vi "Load FIR coeff from CSV.vi"(8 "error in (no error)":T1, 11 "Path":path) -> (0 "error out":T1, 2 "valid":bool, 3 "1D Array":cdb[](array[numeric]))   [LabVIEW 2019]
uses:
  <vilib>/Utility/file.llb/Read Delimited Spreadsheet (string).vi
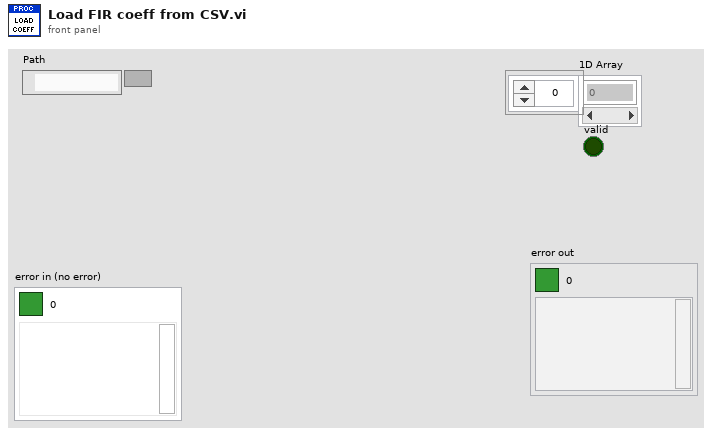
[diagram p1: front panel]
types:
  T1 = cluster{"Boolean Round":bool, "code":i32, "source":string}
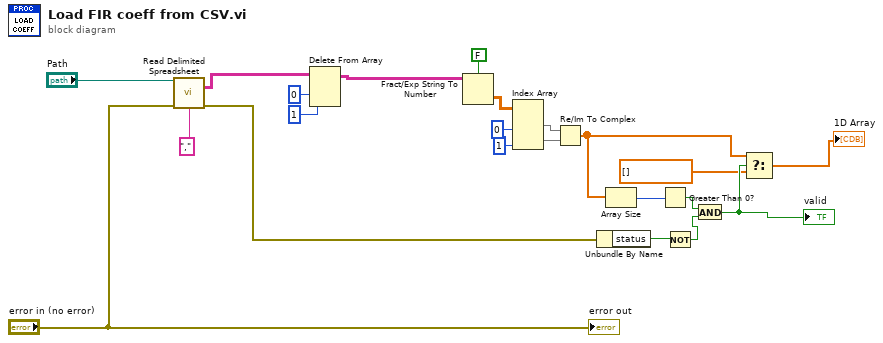
[diagram p0: block diagram]
diagram:
  n1 = call-poly <vilib>:"Read Delimited Spreadsheet.vi"("file path (dialog if empty)"="Path", "error in (no error)"="error in (no error)", "delimiter (\\t)"="," ("delimiter (\\t)")) -> ("all rows"=w20:string[][], "error out"=w8:errorcluster)  [unwired: 7 in, 4 out]
  n2 = Delete From Array(array=w20, length=1, index (row)=0) -> (array with subset deleted=w17:string[][])  [unwired: 1 in, 1 out]
  n3 = Fract/Exp String To Number(use system decimal point (T)=FALSE, string=w17) -> (number=w16:dbl[][])  [unwired: 2 in, 1 out]
  n4 = Index Array(array=w16, index (col) #1=0 ("disabled index (col)"), index (col) #2=1 ("disabled index (col)")) -> (element #1=w13:dbl[], element #2=w12:dbl[])  [unwired: 2 in]
  n5 = Re/Im To Complex(1:w12, 2:w13) -> (0:w4:cdb[])
  n6 = Unbundle By Name(w8) -> ("status"=w7:bool)
  n7 = Array Size(array=w4) -> (size(s)=w9:i32)
  n8 = Greater Than 0?(x=w9) -> (x > 0?=w6:bool)
  n9 = Not(x=w7) -> (.not. x?=w5:bool)
  n10 = And(x=w6, y=w5) -> (x .and. y?=w3:bool)
  "valid" <- w3
  n11 = Select(t=w4, s=w3, f=cdb[] []) -> (s? t:f=→"1D Array":cdb[])
  "error out" <- "error in (no error)"
